vi "Open Report File.vi"(8 "error in (no error)":errorcluster, 11 "Report Interface In":refnum<class "Report Interface.lvclass">) -> (0 "error out":errorcluster, 3 "Report Interface Out":refnum<class "Report Interface.lvclass">)   [LabVIEW 2020, in "Report Interface.lvclass"]
uses:
  Report Interface.lvclass
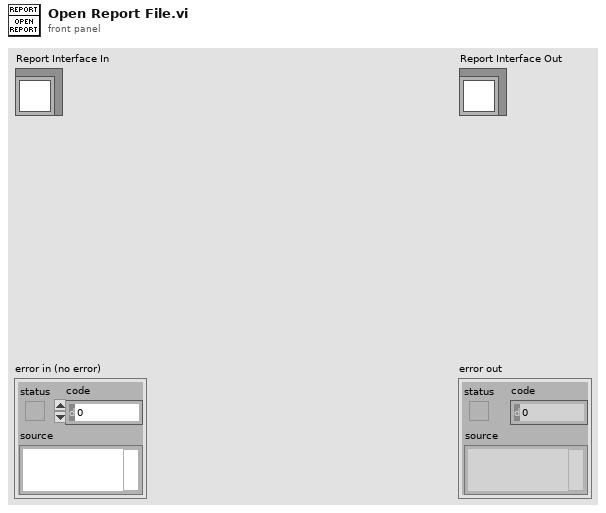
[diagram p1: front panel]
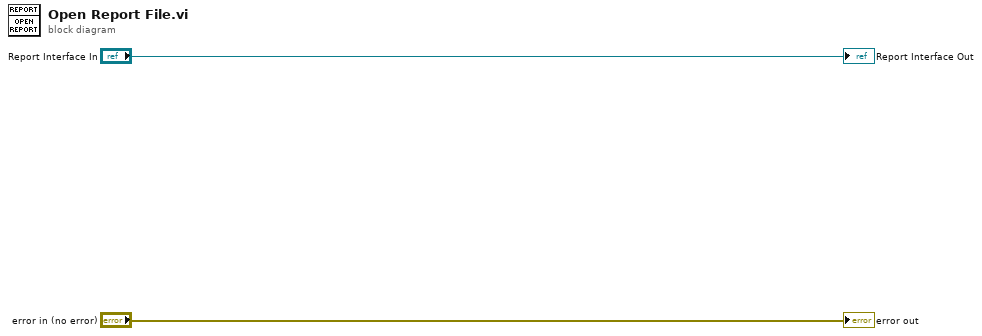
[diagram p0: block diagram]
diagram:
  "error out" <- "error in (no error)"
  "Report Interface Out" <- "Report Interface In"
